vi "MoveBy485.vi"() -> ()   [LabVIEW 2018]
uses:
  <vilib>/robotics/Steering/Create Steering Frame/NI_Robotics_Create Steering Frame.xnode
  <vilib>/robotics/Utilities/Visualization/Steering Visualization/Steering Picture/Draw Steering Frame Options.ctl
  <vilib>/robotics/Steering/Mecanum Steering Frame/NI_Robotics_Mecanum Steering Frame.lvclass
  <vilib>/robotics/Steering/Class Type Definitions/Mecanum Steering Frame.ctl
  XInput9_1_0.dll
  <vilib>/Utility/miscctls.llb/LVPointTypeDef.ctl
  <vilib>/robotics/Steering/Mecanum Steering Frame/Create Mecanum Steering Frame.vi
  <vilib>/robotics/Steering/Mecanum Wheel/Create Mecanum Wheel.vi
  <vilib>/robotics/Steering/Mecanum Wheel/Roller Orientation.ctl
  <vilib>/robotics/Steering/Wheel/Rotation Direction.ctl
  <vilib>/robotics/Steering/Wheel/Wheel Parameters.ctl
  <vilib>/Instr/_visa.llb/VISA Configure Serial Port (Instr).vi
  <vilib>/robotics/Steering/Steering Frame/Apply Steering Frame Velocity to Motors.vi
panel:
  in  "탭 컨트롤":enum32{"Simple", "Setting", "RecipeLab"}(tab)
  out "좌우 속도(m/s)":dbl
  out "회전 속도(rad/s)":dbl
  out "전후 속도(m/s)":dbl
  out "RPM":dbl[](array[numeric])=[0.0, -0.0, 0.0, -0.0]
  in  "Front":bool
  in  "Rear":bool
  in  "Left":bool
  in  "Right":bool
  in  "L Turn":bool
  in  "R Turn":bool
  out "Status":bool
  in  "모터 정지":bool
  out "Motion(Main)":picture caption="Motion"
  in  "최대 전후 속도(m/s)":dbl(slide)=0.1 scale=0.05..0.3
  in  "설정 저장":bool
  in  "최대 좌우 속도(m/s)":dbl(slide)=0.1 scale=0.05..0.3
  in  "최대 회전 속도(rad/s)":dbl(slide)=0.1 scale=0.05..0.3
  in  "RecipeLab 탭 컨트롤":T1(tab)
  in  "Status 유효시간(s)":dbl=0.1
  in  "정지신호 대기시간 (ms)":u32=3000
  out "출력속도(rpm)(recipelab)":dbl[](array[numeric])=[0.0, -0.0, 0.0, -0.0]
  in  "속도제한(rpm)":dbl=2000.0 format="%#_17g"
  in  "속도배율(rpm)":dbl=1.0
  in  "정지":bool
  in  "휠역전":bool[](array[boolean])=[FALSE, FALSE, FALSE, FALSE]
  in  "ID":u8[](array[numeric])=[11, 12, 13, 14]
  in  "Ratio":dbl=50.0 format="%#_13g"
  out "수신 timestamp":timestamp format="%<%H:%M:%S%3u>T"
  out "수신데이터":u8[](array[numeric])
  out "송신데이터":u8[][](array[numeric])
  out "Serial Bytes":u32
  out "송신 timestamp":timestamp=timestamp(3699356400 s since 1904-01-01) format="%<%H:%M:%S%3u>T"
  in  "VISA Write":bool=TRUE
  in  "VISA":refnum<visa-resource-name>="COM7"
  out "송신주기(ms)":u32(graph)=41
  out "수신주기(ms)":u32(graph)
  in  "Angular Velocity (rad/s)":dbl(slide) min=-0.5 max=0.5 step=0.01 scale=-0.1..0.1
  in  "Lateral Velocity (m/s)":dbl(slide) min=-0.5 max=0.5 step=0.01 scale=-0.1..0.1
  in  "Forward Velocity (m/s)":dbl(slide) min=-0.5 max=0.5 step=0.01 scale=-0.1..0.1
  out "Motion(Control)":picture caption="Motion"
  out "출력속도(rpm)(Control)":dbl[](array[numeric])=[0.0, -0.0, 0.0, -0.0]
  out "Buttons":T2
  out "XInput Return":u32
  out "pState":T3
  out "X(Joy)":dbl
  out "Y(Joy)":dbl
  out "Z(Joy)":dbl
  in  "조이스틱 사용":bool
  out "조이스틱 연결됨?":bool
  in  "속도배율(Joy)":dbl=0.05 format="%#_13g"
  out "Motion(Joy)":picture caption="Motion"
  out "출력속도(rpm)(Joystick)":dbl[](array[numeric])=[0.0, -0.0, 0.0, -0.0]
  in  "VISA(str)":string="COM7"
  in  "저장라벨명":string[](array[string])=["저장라벨명", "저장라벨명(str)", "정지신호 대기시간 (ms)", "속도제한(rpm)", "속도배율(rpm)", "휠역전", "VISA Write", "속도배율(Joy)", "ID", "Status 유효시간(s)", "최대 전후 속도(m/s)", "최대 좌우 속도(m/s)", "최대 회전 속도(rad/s)", "Ratio"]
  in  "저장라벨명(str)":string[](array[string])=["VISA(str)"]
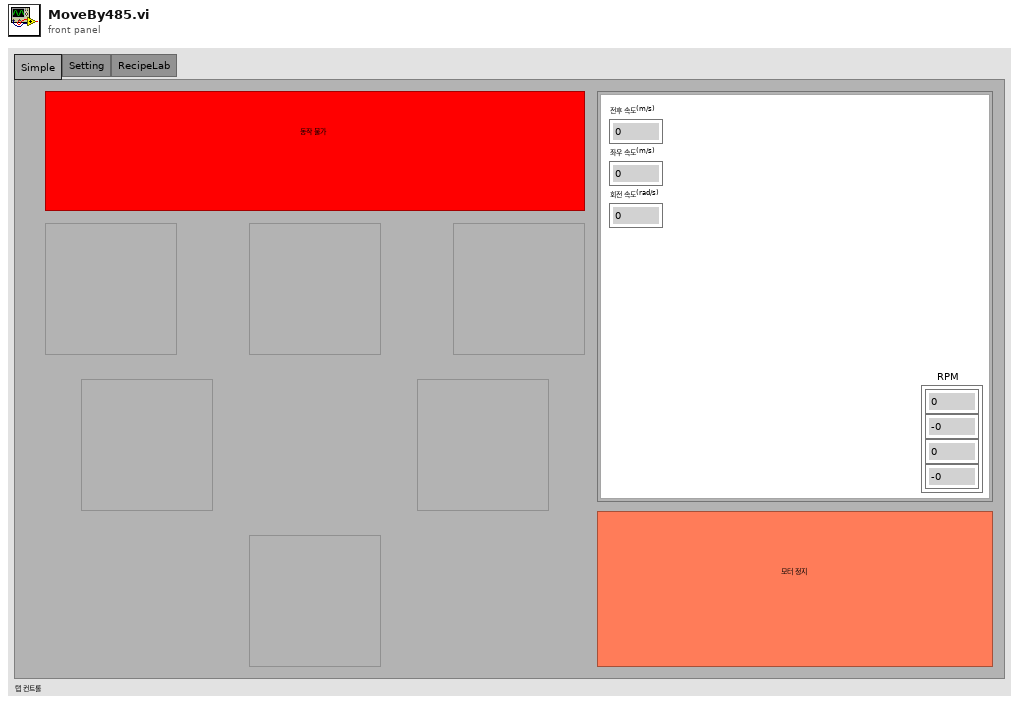
[diagram p1: front panel]
types:
  T1 = enum32{"RecipeLab", "Serial", "Control", "Joystick", "Setting"}
  T2 = cluster{"Dpad Up":bool, "Dpad Down":bool, "Dpad Left":bool, "Dpad Right":bool, "Menu":bool, "View":bool, "L Stick":bool, "R Stick":bool, "L Bumper":bool, "R Bumper":bool, "UNKNOWN":bool, "UNKNOWN":bool, "A":bool, "B":bool, "X":bool, "Y":bool}
  T3 = cluster{"Packet Number":u32, "Gamepad":cluster{"Buttons":u16, "Left Trigger":u8, "Right Trigger":u8, "Thumb LX":i16, "Thumb LY":i16, "Thumb RX":i16, "Thumb RY":i16}}
  T4 = enum32{"invalid app kind", "Development System", "Run Time System", "Student Edition", "Embedded LabVIEW", "Evaluation", "Custom"}
  T5 = typedef "LVPointTypeDef.ctl" = cluster{"Horizontal":i16, "Vertical":i16}
  T6 = cluster{"Boolean array[0]":bool, "Boolean array[1]":bool, "Boolean array[2]":bool, "Boolean array[3]":bool, "Boolean array[4]":bool, "Boolean array[5]":bool, "Boolean array[6]":bool, "Boolean array[7]":bool, "Boolean array[8]":bool, "Boolean array[9]":bool, "Boolean array[10]":bool, "Boolean array[11]":bool, "Boolean array[12]":bool, "Boolean array[13]":bool, "Boolean array[14]":bool, "Boolean array[15]":bool}
  T7 = typedef "NI_Robotics_Steering Picture.lvlib/Draw Steering Frame Options.ctl" = cluster{"draw wheel states?":bool, "highlight wheel index":i32, "pixels per unit":dbl, "draw forward velocity?":bool, "velocity scale":dbl}
  T8 = typedef "LVBoundsTypeDef.ctl" = cluster{"Width":u32, "Height":u32}
  T9 = typedef "NI_Robotics_Steering Class Types.lvlib/Mecanum Steering Frame.ctl" = refnum<class "NI_Robotics_Mecanum Steering Frame.lvclass">
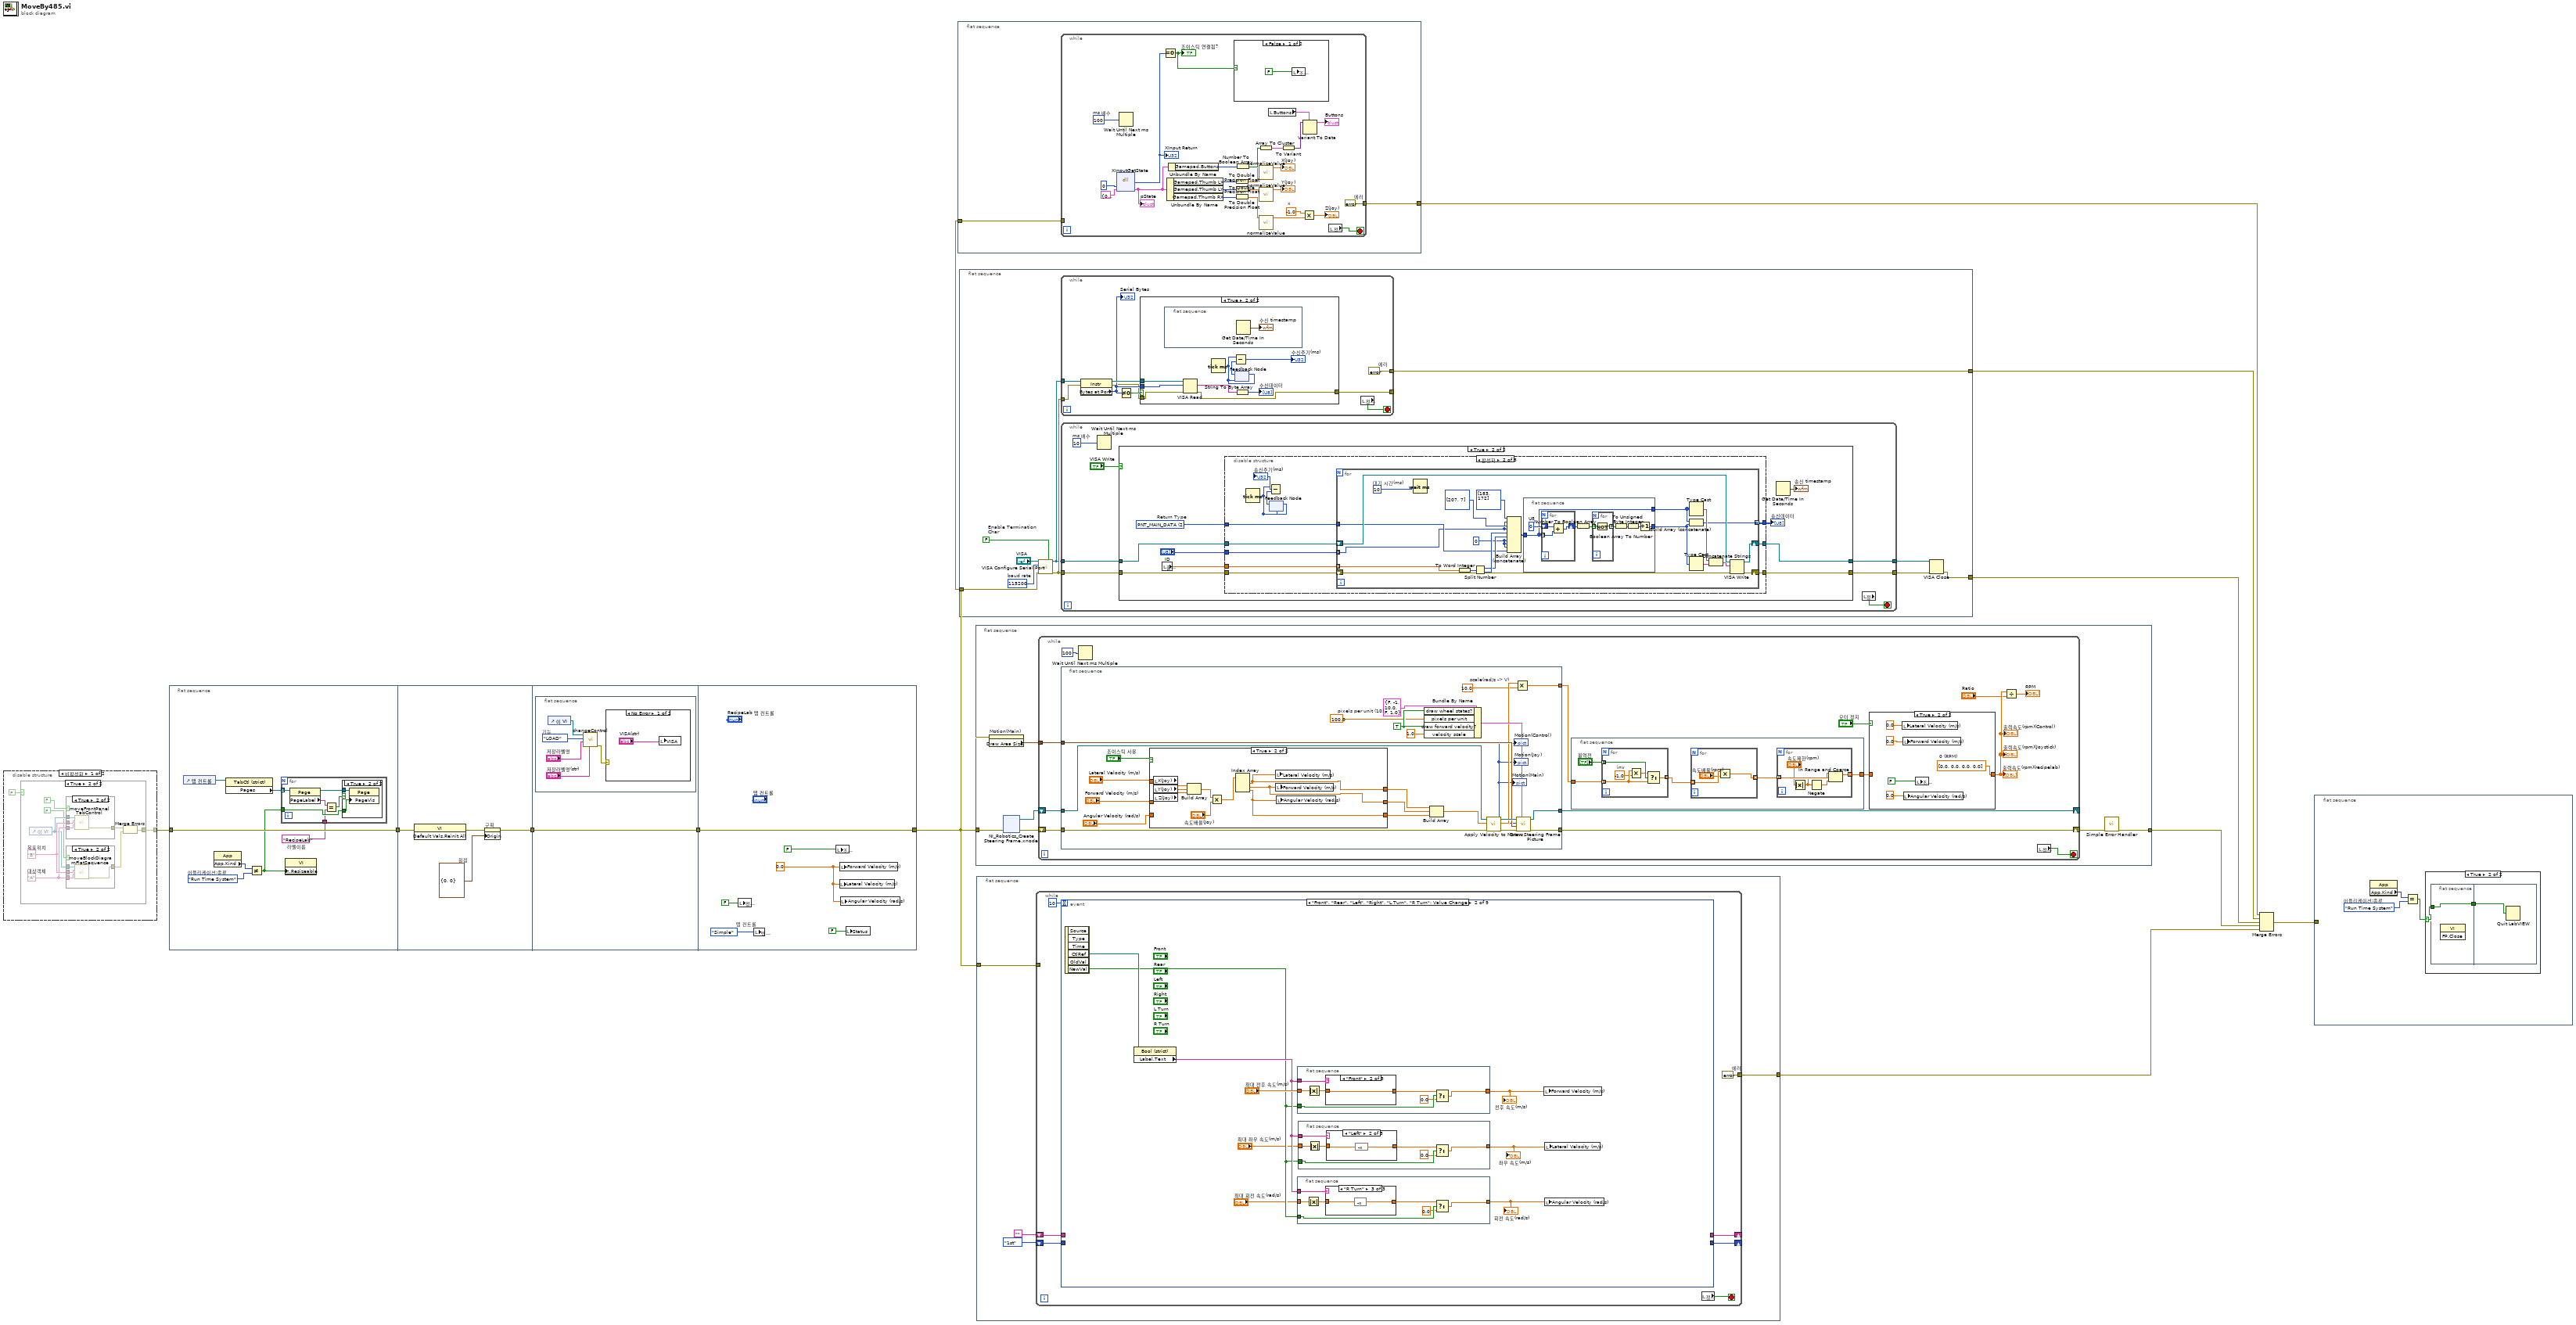
[diagram p0: block diagram]
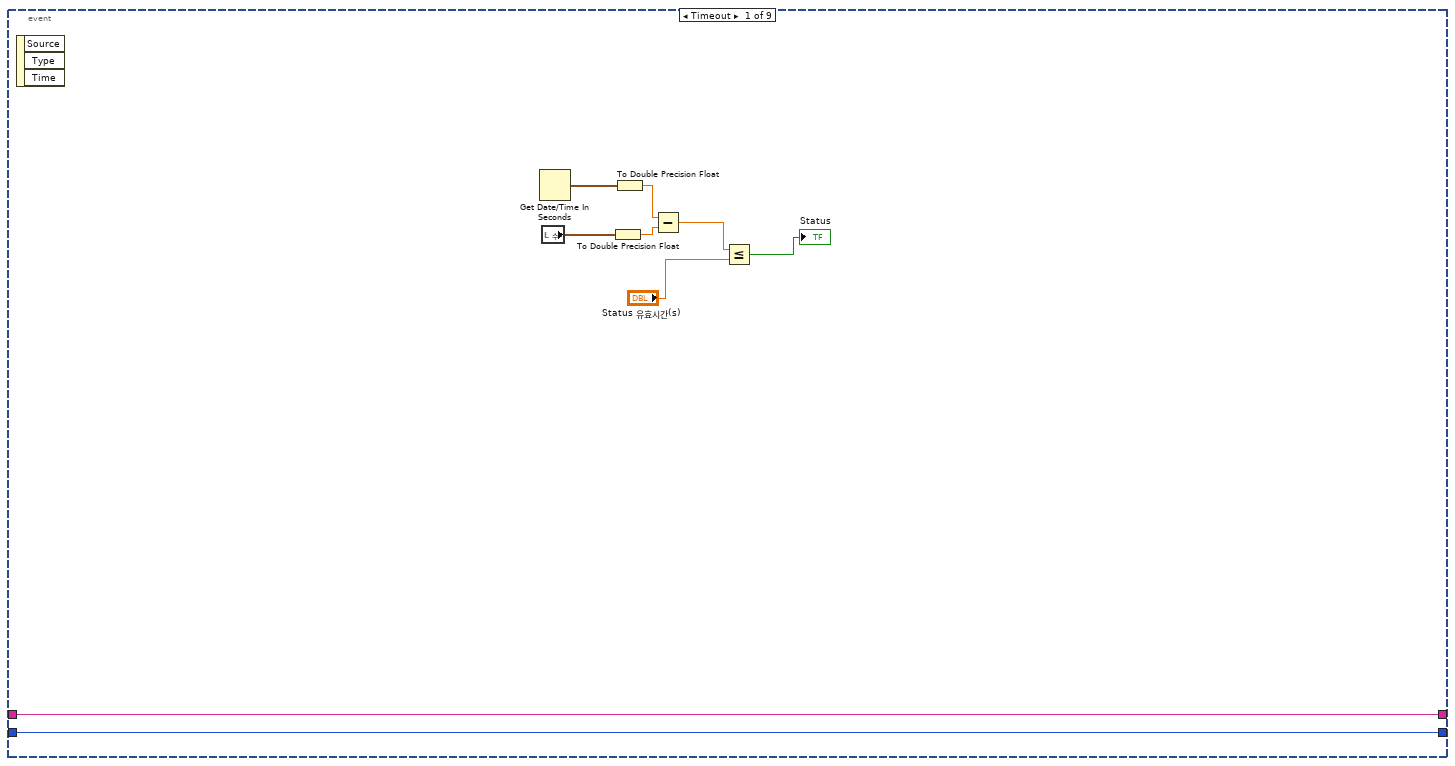
[diagram p2: hidden frame]
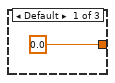
[diagram p3: hidden frame]
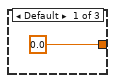
[diagram p5: hidden frame]
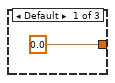
[diagram p7: hidden frame]
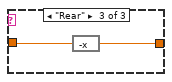
[diagram p8: hidden frame]
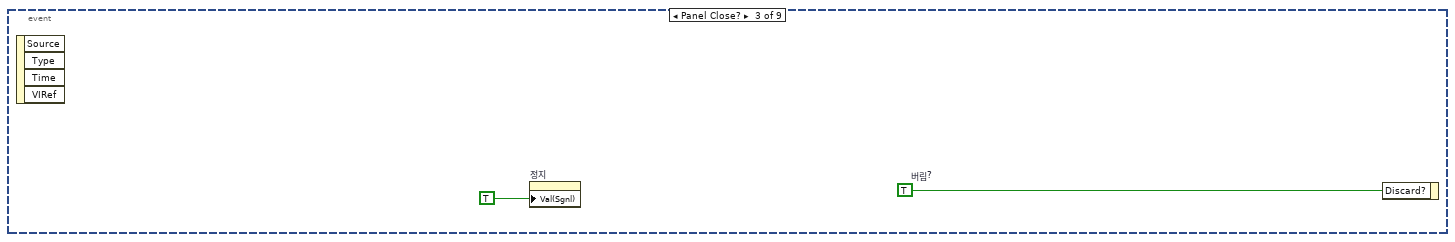
[diagram p9: hidden frame]
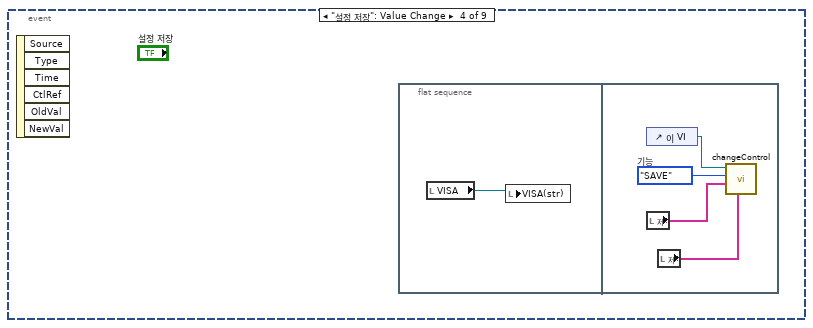
[diagram p10: hidden frame]
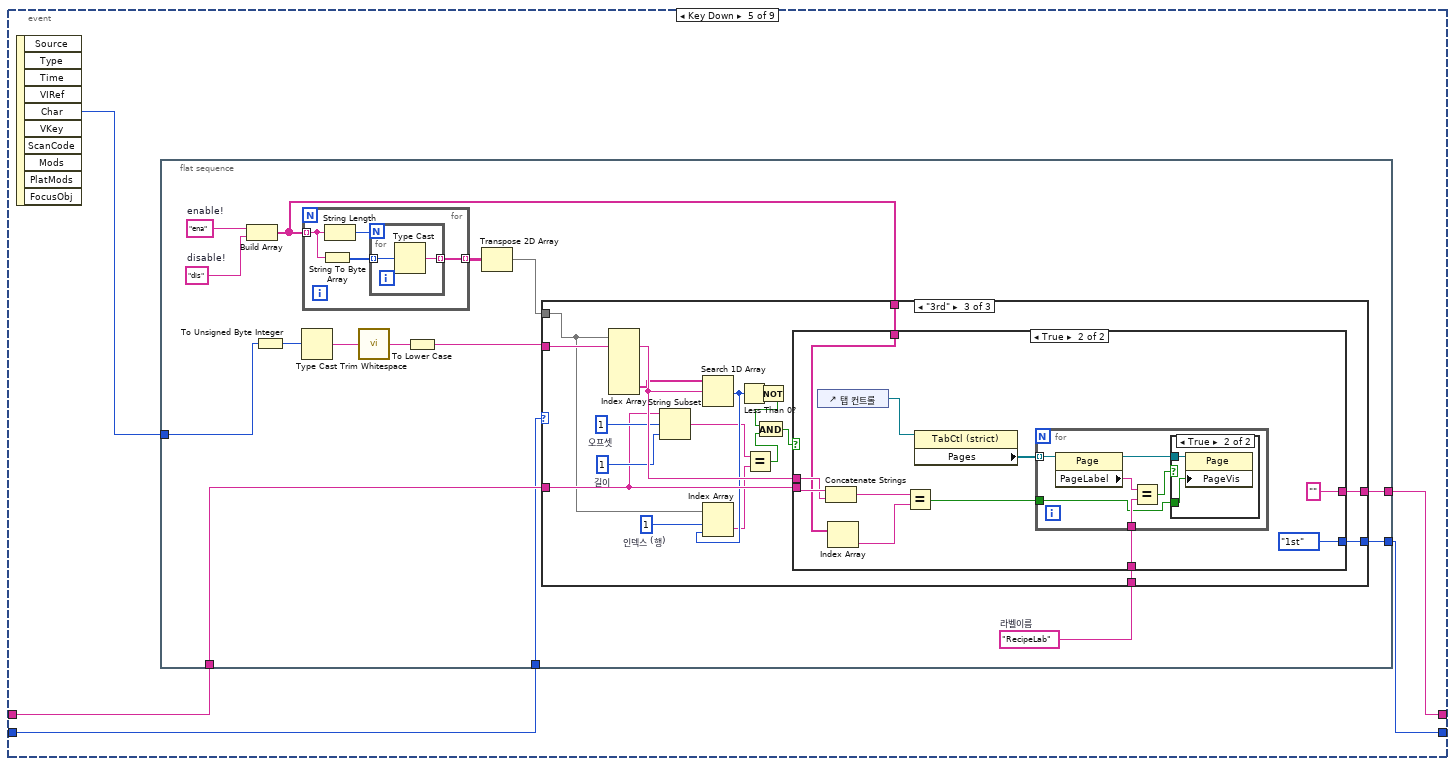
[diagram p11: hidden frame]
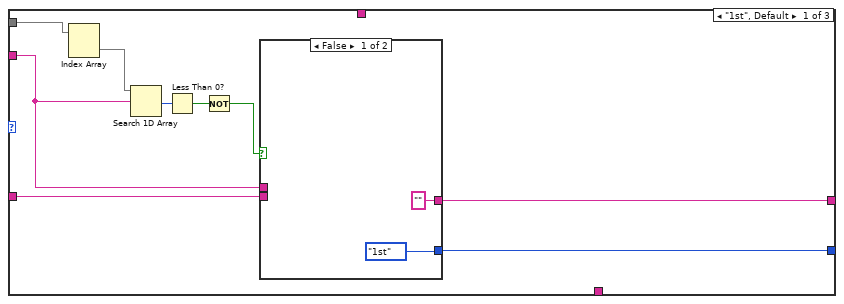
[diagram p12: hidden frame]
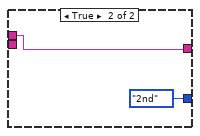
[diagram p13: hidden frame]
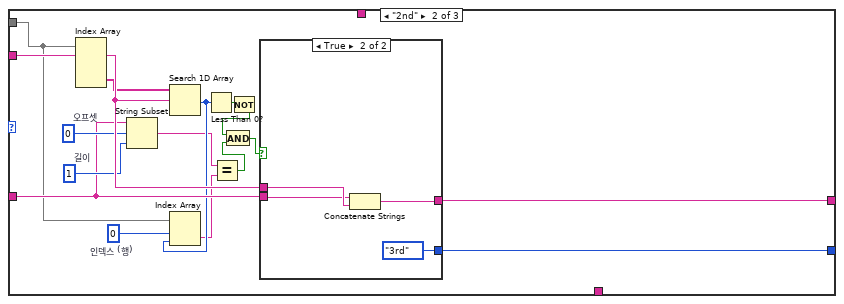
[diagram p14: hidden frame]
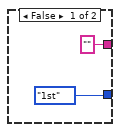
[diagram p15: hidden frame]
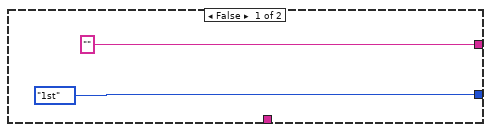
[diagram p16: hidden frame]
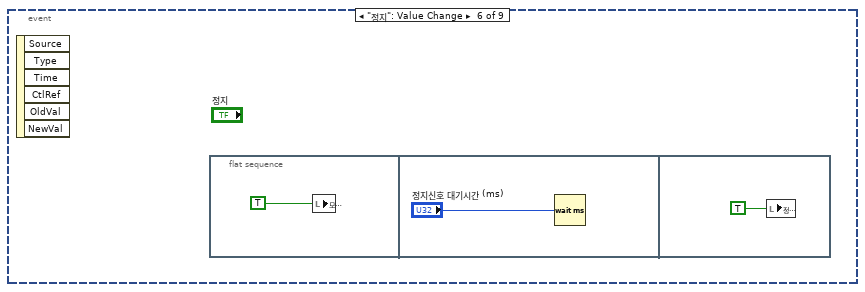
[diagram p18: hidden frame]
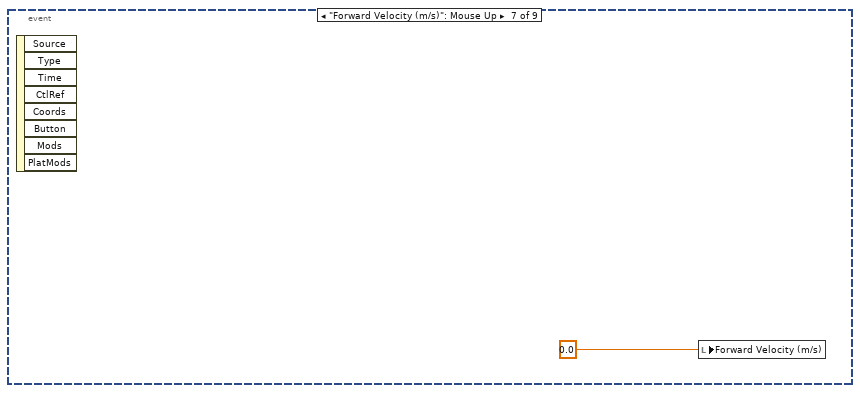
[diagram p19: hidden frame]
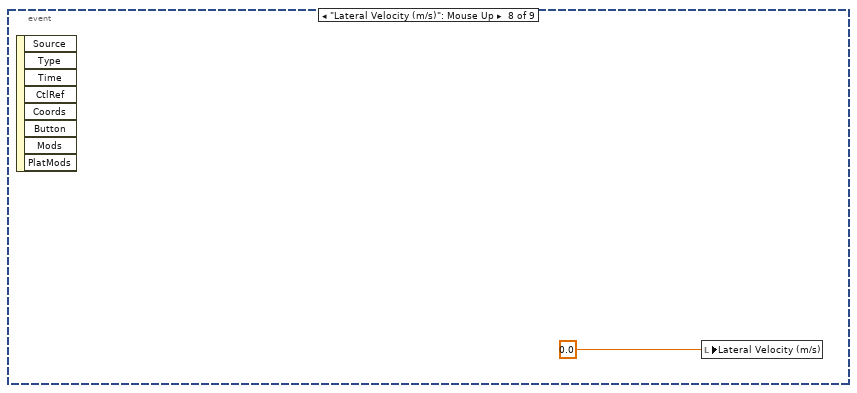
[diagram p20: hidden frame]
diagram:
  n1 = disable-structure shown="비활성화" {
    disable-tunnel: [w12 _] -> w11
    frame Disabled {
      n2 = case shown="True" FALSE {
        tunnel: [_ w14] -> w12
        frame False {
        }
        frame True {
          w20 = "A"  # 대상객체
          w21 = "B"  # 목표위치
          n3 = control-ref of="이 VI"() -> (w19:refnum<vi>)
          n4 = case shown="True" FALSE {
            tunnel: w19 -> [_ w31]
            tunnel: w21 -> [_ w30]
            tunnel: w20 -> [_ w29]
            tunnel: [w27 w28] -> w18
            frame False {
              w27 = errorcluster {"status"=FALSE, "code"=0, "source"=""}  # 에러
            }
            frame True {
              n5 = call "moveFrontPanelTabControl.vi"("대상객체"=w29, "목표위치"=w30, "VI 참조"=w31) -> ("error out"=w28:errorcluster)  [unwired: 7 in, 1 out]
            }
          }
          n6 = case shown="True" FALSE {
            tunnel: w21 -> [_ w26]
            tunnel: w20 -> [_ w25]
            tunnel: w19 -> [_ w24]
            tunnel: [w22 w23] -> w17
            frame False {
              w22 = errorcluster {"status"=FALSE, "code"=0, "source"=""}  # 에러
            }
            frame True {
              n7 = call "moveBlockDiagramFlatSequence.vi"("대상객체"=w25, "목표위치"=w26, "VI 참조"=w24) -> ("error out"=w23:errorcluster)  [unwired: 7 in, 1 out]
            }
          }
          n8 = Merge Errors(w18, w17) -> (w14:errorcluster)
        }
      }
    }
    frame Enabled {
    }
  }
  n9 = flat-sequence {
    tunnel: w11 -> [w38]
    tunnel: [w38] -> w10
    tunnel: [w49] -> w9
    tunnel: w10 -> [w50]
    tunnel: w9 -> [w51]
    tunnel: [w51] -> w8
    tunnel: [w63] -> w3
    tunnel: w8 -> [w63]
    frame #0 {
      w34 = "RecipeLab"  # 라벨이름
      w33 = T4."Run Time System"  # 어플리케이션:종류
      n10 = control-ref of="탭 컨트롤"() -> (w32:refnum<vi>)
      n11 = property class="App"() -> ("App.Kind"=w35:T4)  [unwired: 2 in, 2 out]
      n12 = property class="TabCtl (strict)"(reference=w32) -> ("Pages"=w36:refnum<vi>[])  [unwired: 1 in, 2 out]
      n13 = Not Equal?(x=w35, y=w33) -> (x != y?=w37:bool)
      n14 = for {
        tunnel: w36 -> [w44] mode=indexing
        tunnel: w37 -> [w40]
        tunnel: w34 -> [w39]
        n15 = property class="Page"(reference=w44) -> (reference out=w41:refnum<vi>, "PageLabel"=w43:string)  [unwired: 1 in, 1 out]
        n16 = Equal?(x=w43, y=w39) -> (x = y?=w42:bool)
        n17 = case shown="True" w42 {
          tunnel: w41 -> [_ w46]
          tunnel: w40 -> [_ w45]
          frame False {
          }
          frame True {
            n18 = property class="Page"(reference=w46, "PageVis"=w45) -> ()  [unwired: 1 in, 2 out]
          }
        }
      }
      n19 = property on="프로퍼티 노드" class="VI"("Front Panel.Resizeable"=w37) -> ()  [unwired: 2 in, 2 out]
    }
    frame #1 {
      w48 = T5 {"Horizontal"=0, "Vertical"=0}  # 원점
      n20 = invoke class="VI" method="Default Vals.Reinit All"(error in=w50) -> (error out=w47:errorcluster)  [unwired: 2 in, 2 out]
      n21 = property on="구획" class="Pane"(error in=w47, "Origin"=w48) -> (error out=w49:errorcluster)  [unwired: 1 in, 1 out]
    }
    frame #2 {
      n22 = flat-sequence {
        frame #0 {
          w53 = enum16{"LOAD", "SAVE"}."LOAD"  # 기능
          n23 = control-ref of="이 VI"() -> (w54:refnum<vi>)
          n24 = call "changeControl.vi"("라벨명(str)"="저장라벨명(str)", "라벨명"="저장라벨명", "기능"=w53, "VI 참조"=w54) -> ("error out"=w52:errorcluster)  [unwired: 7 in]
          n25 = case shown="No Error" w52 {
            frame No Error {
              n26 = local write "VISA"("VISA(str)") -> ()
            }
            frame Error {
            }
          }
        }
      }
    }
    frame #3 {
      w59 = 0.0
      w60 = enum32{"Simple", "Setting", "RecipeLab"}."Simple"  # 탭 컨트롤
      n27 = local write "정지"(FALSE) -> ()
      n28 = local write "탭 컨트롤"(w60) -> ()
      n29 = local write "조이스틱 사용"(FALSE) -> ()
      n30 = local write "Lateral Velocity (m/s)"(w59) -> ()
      n31 = local write "Forward Velocity (m/s)"(w59) -> ()
      n32 = local write "Angular Velocity (rad/s)"(w59) -> ()
      n33 = local write "Status"(FALSE) -> ()
    }
  }
  n34 = flat-sequence {
    tunnel: w3 -> [w65]
    tunnel: [w64] -> w7
    frame #0 {
      n35 = while {
        tunnel: w65 -> [_]
        tunnel: [w67] -> w64
        stop <- w73 stop-if-true
        w67 = errorcluster {"status"=FALSE, "code"=0, "source"=""}  # 에러
        w68 = -1.0  # x
        w90 = u32 100  # ms 배수
        n36 = dll-call lib="XInput9_1_0.dll" fn="XInputGetState"("dwUserIndex"=u32 0, "pState"=T3 {"Packet Number"=0, "Gamepad"={"Buttons"=0, "Left Trigger"=0, "Right Trigger"=0, "Thumb LX"=0, "Thumb LY"=0, "Thumb RX"=0, "Thumb RY"=0}} ("XInput State")) -> ("return type"=w82:u32, "pState"=w80:T3)  [unwired: 4 in, 2 out]
        "XInput Return" <- w82
        "pState" <- w80
        n37 = Wait Until Next ms Multiple(millisecond multiple=w90) -> ()  [unwired: 1 out]
        n38 = Equal To 0?(x=w82) -> (x = 0?=w66:bool)
        "조이스틱 연결됨?" <- w66
        n39 = Unbundle By Name(w80) -> ("Gamepad.Thumb LX"=w79:i16, "Gamepad.Thumb LY"=w76:i16, "Gamepad.Thumb RX"=w70:i16)
        n40 = Unbundle By Name(w80) -> ("Gamepad.Buttons"=w85:u16)
        n41 = case shown="False" w66 {
          frame False {
            n42 = local write "조이스틱 사용"(FALSE) -> ()
          }
          frame True {
          }
        }
        n43 = To Double Precision Float(number=w79) -> (double precision float=w78:dbl)
        n44 = To Double Precision Float(number=w76) -> (double precision float=w75:dbl)
        n45 = To Double Precision Float(number=w70) -> (double precision float=w71:dbl)
        n46 = Number To Boolean Array(number=w85) -> (Boolean array=w83:bool[])
        n47 = Array To Cluster(array=w83) -> (cluster=w89:T6)
        n48 = call "normalizeValue.vi"("입력"=w78) -> ("출력"=→"X(Joy)":dbl)  [unwired: 9 in, 1 out]
        n49 = call "normalizeValue.vi"("입력"=w75) -> ("출력"=→"Y(Joy)":dbl)  [unwired: 9 in, 1 out]
        n50 = call "normalizeValue.vi"("입력"=w71) -> ("출력"=w72:dbl)  [unwired: 9 in, 1 out]
        n51 = local read "Buttons"() -> (w84:T2)
        n52 = To Variant(anything=w89) -> (Variant=w88:variant)
        n53 = Multiply(x=w68, y=w72) -> (x*y=→"Z(Joy)":dbl)
        n54 = Variant To Data(type=w84, Variant=w88) -> (data=→"Buttons":T2)  [unwired: 1 in, 1 out]
        n55 = local read "정지"() -> (w73:bool)
      }
    }
  }
  n56 = flat-sequence {
    tunnel: w3 -> [w96]
    tunnel: [w95] -> w6
    tunnel: [w92] -> w2
    frame #0 {
      w99 = FALSE  # Enable Termination Char
      w100 = u32 115200  # baud rate
      n57 = call-poly "VISA Configure Serial Port"("VISA resource name"="VISA", "Enable Termination\nChar (T)"=w99, "baud rate (9600)"=w100, "error in (no error)"=w96) -> ("VISA resource name out"=w97:refnum<visa-resource-name>, "error out"=w98:errorcluster)  [unwired: 10 in]
      n58 = while {
        tunnel: w98 -> [w105]
        tunnel: w97 -> [w109]
        tunnel: [w103] -> _
        tunnel: [w102] -> w95
        stop <- w106 stop-if-true
        w102 = errorcluster {"status"=FALSE, "code"=0, "source"=""}  # 에러
        n59 = property class="Instr"(reference=w109, error in=w105) -> (reference out=w110:refnum<visa-resource-name>, error out=w104:errorcluster, "Bytes at Port"=w107:u32)
        "Serial Bytes" <- w107
        n60 = Not Equal To 0?(x=w107) -> (x != 0?=w108:bool)
        n61 = case shown="True" w108 {
          tunnel: w110 -> [_ w120]
          tunnel: w107 -> [_ w119]
          tunnel: w104 -> [w111 w113]
          tunnel: [w111 w112] -> w103
          frame False {
          }
          frame True {
            n62 = flat-sequence {
              frame #0 {
                n63 = Get Date/Time In Seconds() -> (seconds since 1Jan1904=→"수신 timestamp":timestamp)
              }
            }
            n64 = VISA Read(VISA resource name=w120, byte count=w119, error in (no error)=w113) -> (read buffer=w118:string, error out=w112:errorcluster)  [unwired: 2 out]
            n65 = Tick Count (ms)() -> (millisecond timer value=w115:u32)
            n66 = feedback-in #1(w115) -> ()
            n67 = feedback #1(w115) -> (w116:u32)
            n68 = Subtract(x=w115, y=w116) -> (x-y=→"수신주기(ms)":u32)
            n69 = String To Byte Array(string=w118) -> (unsigned byte array=→"수신데이터":u8[])
          }
        }
        n70 = local read "정지"() -> (w106:bool)
      }
      n71 = while {
        tunnel: w97 -> [w128]
        tunnel: [w124] -> w93
        tunnel: [w123] -> w94
        tunnel: w98 -> [w126]
        stop <- w122 stop-if-true
        w125 = u32 10  # ms 배수
        n72 = Wait Until Next ms Multiple(millisecond multiple=w125) -> ()  [unwired: 1 out]
        n73 = case shown="True" "VISA Write" {
          tunnel: w128 -> [w130 w139]
          tunnel: [w130 w138] -> w124
          tunnel: [w129 w137] -> w123
          tunnel: w126 -> [w129 w136]
          frame False {
          }
          frame True {
            w132 = u8 2 items=["No Return", "PNT_MONITOR", "PNT_MAIN_DATA"]  # Return Type
            n74 = local read "출력속도(rpm)(recipelab)"() -> (w133:dbl[])
            n75 = disable-structure shown="활성화" {
              disable-tunnel: w139 -> [w154 w205 w246]
              disable-tunnel: [w153 w204 w245] -> w138
              disable-tunnel: [w152 w203 w244] -> w137
              disable-tunnel: w136 -> [w151 w202 w243]
              disable-tunnel: "ID" -> [w144 w199 w242]
              disable-tunnel: [w150 w201 w241] -> w134
              disable-tunnel: w133 -> [w143 w200 w240]
              disable-tunnel: w132 -> [w140 w198 _]
              frame Disabled {
                w145 = 2 ("인덱스")
                n76 = Split 1D Array(array=w144, index=w145) -> (first subarray=w146:u8[], second subarray=w147:u8[])
                n77 = Split 1D Array(array=w143, index=w145) -> (first subarray=w148:dbl[], second subarray=w149:dbl[])
                n78 = Build Array(w146, w147) -> (w142:u8[][])
                n79 = Build Array(w148, w149) -> (w141:dbl[][])
                n80 = for {
                  shift-right: [w180] -> w153
                  shift-left: w154 -> [w181]
                  shift-right: [w179] -> w152
                  shift-left: w151 -> [w178]
                  tunnel: w141 -> [w156] mode=indexing
                  tunnel: w142 -> [w157] mode=indexing
                  tunnel: [w173] -> w150 mode=indexing
                  tunnel: w140 -> [w155]
                  w174 = u32 10  # 대기 시간(ms)
                  n81 = Wait (ms)(milliseconds to wait=w174) -> ()  [unwired: 1 out]
                  n82 = Index Array(array=w156) -> (element #1=w166:dbl, element #2=w170:dbl)  [unwired: 2 in]
                  n83 = To Word Integer(number=w166) -> (16bit integer=w165:i16)
                  n84 = To Word Integer(number=w170) -> (16bit integer=w169:i16)
                  n85 = Index Array(array=w157) -> (element #1=w167:u8, element #2=w168:u8)  [unwired: 2 in]
                  n86 = Split Number(x=w165) -> (hi(x)=w162:u8, lo(x)=w163:u8)
                  n87 = Split Number(x=w169) -> (hi(x)=w172:u8, lo(x)=w171:u8)
                  n88 = Build Array (concatenate)(u8[] [183, 172, 254] ("velocity command"), u8[] [207, 7] ("velocity command"), w167, w163, w162, w168, w171, w172, w155) -> (w164:u8[])
                  n89 = flat-sequence {
                    tunnel: [w183] -> w158
                    tunnel: w164 -> [w182]
                    tunnel: [w182] -> w159
                    frame #0 {
                      w189 = u8 0  # U8
                      n90 = for {
                        tunnel: w182 -> [w193] mode=indexing
                        shift-right: [w192] -> w188
                        shift-left: w189 -> [w194]
                        n91 = Add(x=w194, y=w193) -> (x+y=w192:u8)
                      }
                      n92 = Number To Boolean Array(number=w188) -> (Boolean array=w187:bool[])
                      n93 = for {
                        tunnel: w187 -> [w191] mode=indexing
                        tunnel: [w190] -> w186 mode=indexing
                        n94 = Not(x=w191) -> (.not. x?=w190:bool)
                      }
                      n95 = Boolean Array To Number(Boolean array=w186) -> (number=w185:u8)
                      n96 = To Unsigned Byte Integer(number=w185) -> (unsigned 8bit integer=w184:u8)
                      n97 = Increment(x=w184) -> (x+1=w183:u8)
                    }
                  }
                  n98 = Type Cast(x=w159) -> (*(type *) &x=w175:string)  [unwired: 1 in]
                  n99 = Build Array (concatenate)(w159, w158) -> (w173:u8[])
                  n100 = Type Cast(x=w158) -> (*(type *) &x=w177:string)  [unwired: 1 in]
                  n101 = Concatenate Strings(w175, w177) -> (w176:string)
                  n102 = VISA Write(VISA resource name=w181, write buffer=w176, error in (no error)=w178) -> (VISA resource name out=w180:refnum<visa-resource-name>, error out=w179:errorcluster)  [unwired: 1 out]
                }
              }
              frame Enabled {
                n103 = Tick Count (ms)() -> (millisecond timer value=w196:u32)
                n104 = feedback #2(w196) -> (w195:u32)
                n105 = Subtract(x=w196, y=w195) -> (x-y=→"송신주기(ms)":u32)
                n106 = feedback-in #2(w196) -> ()
                n107 = for {
                  shift-right: [w225] -> w204
                  shift-left: w205 -> [w226]
                  shift-right: [w224] -> w203
                  shift-left: w202 -> [w223]
                  tunnel: w200 -> [w208] mode=indexing
                  tunnel: w199 -> [w207] mode=indexing
                  tunnel: [w218] -> w201 mode=indexing
                  tunnel: w198 -> [w209]
                  w206 = u8 0
                  w219 = u32 10  # 대기 시간(ms)
                  n108 = Wait (ms)(milliseconds to wait=w219) -> ()  [unwired: 1 out]
                  n109 = To Word Integer(number=w208) -> (16bit integer=w217:i16)
                  n110 = Split Number(x=w217) -> (hi(x)=w214:u8, lo(x)=w215:u8)
                  n111 = Build Array (concatenate)(u8[] [183, 172] ("velocity command"), w207, u8[] [207, 7] ("velocity command"), w207, w215, w214, w206, w206, w206, w209) -> (w216:u8[])
                  n112 = flat-sequence {
                    tunnel: [w228] -> w210
                    tunnel: w216 -> [w227]
                    tunnel: [w227] -> w211
                    frame #0 {
                      w234 = u8 0  # U8
                      n113 = for {
                        tunnel: w227 -> [w238] mode=indexing
                        shift-right: [w237] -> w233
                        shift-left: w234 -> [w239]
                        n114 = Add(x=w239, y=w238) -> (x+y=w237:u8)
                      }
                      n115 = Number To Boolean Array(number=w233) -> (Boolean array=w232:bool[])
                      n116 = for {
                        tunnel: w232 -> [w236] mode=indexing
                        tunnel: [w235] -> w231 mode=indexing
                        n117 = Not(x=w236) -> (.not. x?=w235:bool)
                      }
                      n118 = Boolean Array To Number(Boolean array=w231) -> (number=w230:u8)
                      n119 = To Unsigned Byte Integer(number=w230) -> (unsigned 8bit integer=w229:u8)
                      n120 = Increment(x=w229) -> (x+1=w228:u8)
                    }
                  }
                  n121 = Type Cast(x=w211) -> (*(type *) &x=w220:string)  [unwired: 1 in]
                  n122 = Build Array (concatenate)(w211, w210) -> (w218:u8[])
                  n123 = Type Cast(x=w210) -> (*(type *) &x=w222:string)  [unwired: 1 in]
                  n124 = Concatenate Strings(w220, w222) -> (w221:string)
                  n125 = VISA Write(VISA resource name=w226, write buffer=w221, error in (no error)=w223) -> (VISA resource name out=w225:refnum<visa-resource-name>, error out=w224:errorcluster)  [unwired: 1 out]
                }
              }
              frame Disabled {
                n126 = for {
                  shift-right: [w264] -> w245
                  shift-left: w246 -> [w265]
                  shift-right: [w263] -> w244
                  shift-left: w243 -> [w262]
                  tunnel: w240 -> [w255] mode=indexing
                  tunnel: w242 -> [w251] mode=indexing
                  tunnel: [w247] -> w241 mode=indexing
                  w250 = u32 10  # 대기 시간(ms)
                  w252 = u8[] [130, 2]  # velocity command
                  w253 = u8[] [183, 172]  # velocity command
                  n127 = To Word Integer(number=w255) -> (16bit integer=w254:i16)
                  n128 = Wait (ms)(milliseconds to wait=w250) -> ()  [unwired: 1 out]
                  n129 = Split Number(x=w254) -> (hi(x)=w259:u8, lo(x)=w258:u8)
                  n130 = Build Array (concatenate)(w253, w251, w252, w258, w259) -> (w257:u8[])
                  n131 = flat-sequence {
                    tunnel: [w267] -> w248
                    tunnel: w257 -> [w266]
                    tunnel: [w266] -> w249
                    frame #0 {
                      w273 = u8 0  # U8
                      n132 = for {
                        tunnel: w266 -> [w277] mode=indexing
                        shift-right: [w276] -> w272
                        shift-left: w273 -> [w278]
                        n133 = Add(x=w278, y=w277) -> (x+y=w276:u8)
                      }
                      n134 = Number To Boolean Array(number=w272) -> (Boolean array=w271:bool[])
                      n135 = for {
                        tunnel: w271 -> [w275] mode=indexing
                        tunnel: [w274] -> w270 mode=indexing
                        n136 = Not(x=w275) -> (.not. x?=w274:bool)
                      }
                      n137 = Boolean Array To Number(Boolean array=w270) -> (number=w269:u8)
                      n138 = To Unsigned Byte Integer(number=w269) -> (unsigned 8bit integer=w268:u8)
                      n139 = Increment(x=w268) -> (x+1=w267:u8)
                    }
                  }
                  n140 = Type Cast(x=w249) -> (*(type *) &x=w256:string)  [unwired: 1 in]
                  n141 = Build Array (concatenate)(w249, w248) -> (w247:u8[])
                  n142 = Type Cast(x=w248) -> (*(type *) &x=w261:string)  [unwired: 1 in]
                  n143 = Concatenate Strings(w256, w261) -> (w260:string)
                  n144 = VISA Write(VISA resource name=w265, write buffer=w260, error in (no error)=w262) -> (VISA resource name out=w264:refnum<visa-resource-name>, error out=w263:errorcluster)  [unwired: 1 out]
                }
              }
            }
            "송신데이터" <- w134
            n145 = Get Date/Time In Seconds() -> (seconds since 1Jan1904=→"송신 timestamp":timestamp)
          }
        }
        n146 = local read "정지"() -> (w122:bool)
      }
      n147 = VISA Close(VISA resource name=w93, error in (no error)=w94) -> (error out=w92:errorcluster)
    }
  }
  n148 = flat-sequence {
    tunnel: w3 -> [w281]
    tunnel: [w279] -> w1
    frame #0 {
      n149 = property on="Motion(Main)" class="Pict"(error in=w281) -> ("Draw Area Size"=w284:T8)  [unwired: 1 in, 2 out]
      n150 = xnode ("NI_Robotics_Create Steering Frame.xnode")("error in (no error)"=w281) -> ("mecanum steering frame out"=w283:T9, "error out"=w282:errorcluster)
      n151 = while {
        shift-right: [w320] -> _
        shift-left: w283 -> [w322]
        shift-right: [w318] -> w280
        shift-left: w282 -> [w321]
        tunnel: w284 -> [w319]
        stop <- w314 stop-if-true
        n152 = flat-sequence {
          tunnel: w322 -> [w352]
          tunnel: w321 -> [w351]
          tunnel: [w350] -> w320
          tunnel: w319 -> [w347]
          tunnel: [w341] -> w318
          tunnel: [w338] -> w317
          frame #0 {
            w343 = 100.0  # pixels per unit (10)
            w339 = 10.0  # scale(rad/s -> V)
            w344 = TRUE ("draw wheel states")
            n153 = case shown="True" "조이스틱 사용" {
              tunnel: [w356 w360] -> w335
              tunnel: "Lateral Velocity (m/s)" -> [w356 _]
              tunnel: [w355 w359] -> w333
              tunnel: "Forward Velocity (m/s)" -> [w355 _]
              tunnel: [w354 w357] -> w331
              tunnel: "Angular Velocity (rad/s)" -> [w354 _]
              frame False {
              }
              frame True {
                n154 = local read "X(Joy)"() -> (w364:dbl)
                n155 = local read "Y(Joy)"() -> (w365:dbl)
                n156 = local read "Z(Joy)"() -> (w358:dbl)
                n157 = Build Array(w364, w365, w358) -> (w363:dbl[])
                n158 = Multiply(x=w363, y="속도배율(Joy)") -> (x*y=w361:dbl[])
                n159 = Index Array(array=w361) -> (element #1=w360:dbl, element #2=w359:dbl, element #3=w357:dbl)  [unwired: 3 in]
                n160 = local write "Lateral Velocity (m/s)"(w360) -> ()
                n161 = local write "Forward Velocity (m/s)"(w359) -> ()
                n162 = local write "Angular Velocity (rad/s)"(w357) -> ()
              }
            }
            n163 = Bundle By Name(cluster=T7 {"draw wheel states?"=FALSE, "highlight wheel index"=-1, "pixels per unit"=10.0, "draw forward velocity?"=FALSE, "velocity scale"=1.0} ("draw options"), "draw wheel states?"=w344, "pixels per unit"=w343, "draw forward velocity?"=w344, "velocity scale"=1.0 ("velocity scale (1)")) -> (w342:T7)
            n164 = Build Array(w335, w333, w331) -> (w353:dbl[])
            n165 = call-poly <vilib>:"Apply Velocity to Motors.vi"("error in (no error)"=w351, "steering frame velocity"=w353, "steering frame in"=w352) -> ("error out"=w348:errorcluster, "ccw motor velocity setpoints"=w340:dbl[], "steering frame out"=w349:T9)  [unwired: 4 in, 2 out]
            n166 = Multiply(x=w340, y=w339) -> (x*y=w338:dbl[])
            n167 = call <vilib>:"Draw Steering Frame Picture.vi"("drawing options"=w342, "error in (no error)"=w348, "picture draw area size (pixels)"=w347, "steering frame in"=w349) -> ("error out"=w341:errorcluster, "picture out"=→"Motion(Main)" →"Motion(Joy)" →"Motion(Control)":picture, "steering frame out"=w350:T9)  [unwired: 5 in]
          }
        }
        n168 = Wait Until Next ms Multiple(millisecond multiple=u32 100) -> ()  [unwired: 1 out]
        n169 = flat-sequence {
          tunnel: w317 -> [w369]
          tunnel: [w368] -> w315
          frame #0 {
            n170 = for {
              tunnel: "휠역전" -> [w378] mode=indexing
              tunnel: w369 -> [w376] mode=indexing
              tunnel: [w375] -> w367 mode=indexing
              w374 = -1.0  # inv
              n171 = Multiply(x=w376, y=w374) -> (x*y=w377:dbl)
              n172 = Select(t=w377, s=w378, f=w376) -> (s? t:f=w375:dbl)
            }
            n173 = for {
              tunnel: w367 -> [w373] mode=indexing
              tunnel: [w372] -> w366 mode=indexing
              n174 = Multiply(x=w373, y="속도배율(rpm)") -> (x*y=w372:dbl)
            }
            n175 = for {
              tunnel: w366 -> [w383] mode=indexing
              tunnel: [w382] -> w368 mode=indexing
              n176 = Absolute Value(x="속도제한(rpm)") -> (abs(x)=w380:dbl)
              n177 = Negate(x=w380) -> (-x=w379:dbl)
              n178 = In Range and Coerce(upper limit=w380, x=w383, lower limit=w379) -> (coerced(x)=w382:dbl)  [unwired: 1 out]
            }
          }
        }
        n179 = case shown="True" "모터 정지" {
          tunnel: [w324 w329] -> w313
          tunnel: w315 -> [w324 _]
          frame False {
          }
          frame True {
            w329 = dbl[] [0.0, 0.0, 0.0, 0.0]  # 0 (RPM)
            n180 = local write "Lateral Velocity (m/s)"(0.0) -> ()
            n181 = local write "Forward Velocity (m/s)"(0.0) -> ()
            n182 = local write "Angular Velocity (rad/s)"(0.0) -> ()
            n183 = local write "조이스틱 사용"(FALSE ("조이스틱 사용")) -> ()
          }
        }
        "출력속도(rpm)(recipelab)" <- w313
        "출력속도(rpm)(Joystick)" <- w313
        "출력속도(rpm)(Control)" <- w313
        n184 = Divide(x=w313, y="Ratio") -> (x/y=→"RPM":dbl[])
        n185 = local read "정지"() -> (w314:bool)
      }
      n186 = call <vilib>:"Simple Error Handler.vi"("error in (no error)"=w280) -> ("error out"=w279:errorcluster)  [unwired: 4 in, 4 out]
    }
  }
  n187 = flat-sequence {
    tunnel: [w387] -> w5
    tunnel: w3 -> [w386]
    frame #0 {
      n188 = while {
        tunnel: w386 -> [_]
        shift-right: [w390] -> _
        shift-left: "" -> [w392]
        shift-right: [w389] -> _
        shift-left: enum16{"1st", "2nd", "3rd"}."1st" -> [w391]
        tunnel: [w388] -> w387
        stop <- w394 stop-if-true
        w388 = errorcluster {"status"=FALSE, "code"=0, "source"=""}  # 에러
        n189 = event shown="[1] \"Front\", \"Rear\", \"Left\", \"Right\", \"L Turn\", \"R Turn\": Value Change" {
          selector: _ -> [_ _ _ _ _ _ _ _ _]
          dyn-events: _ -> [_ _ _ _ _ _ _ _ _]
          timeout: 10 -> [_ _ _ _ _ _ _ _ _]
          tunnel: w392 -> [w403 _ _ _ w456 _ _ _ _]
          tunnel: w391 -> [w402 _ _ _ w455 _ _ _ _]
          tunnel: [w403 _ _ _ w454 _ _ _ _] -> w390
          tunnel: [w402 _ _ _ w453 _ _ _ _] -> w389
          event Timeout {
            n190 = event-data() -> ()  [unwired: 1 in, 3 out]
            n191 = Get Date/Time In Seconds() -> (seconds since 1Jan1904=w401:timestamp)
            n192 = local read "수신 timestamp"() -> (w400:timestamp)
            n193 = To Double Precision Float(number=w400) -> (double precision float=w398:dbl)
            n194 = To Double Precision Float(number=w401) -> (double precision float=w399:dbl)
            n195 = Subtract(x=w399, y=w398) -> (x-y=w397:dbl)
            n196 = Less Or Equal?(x=w397, y="Status 유효시간(s)") -> (x <= y?=→"Status":bool)
          }
          event "Front", "Rear", "Left", "Right", "L Turn", "R Turn": Value Change {
            n197 = event-data() -> ("CtlRef"=w412:refnum<vi>, "NewVal"=w406:bool)  [unwired: 1 in, 4 out]
            n198 = property class="Bool (strict)"(reference=w412) -> ("Label.Text"=w407:string)  [unwired: 1 in, 2 out]
            n199 = flat-sequence {
              tunnel: w407 -> [w419]
              tunnel: "최대 회전 속도(rad/s)" -> [w418]
              tunnel: [w414] -> w408
              tunnel: w406 -> [w416]
              frame #0 {
                n200 = Absolute Value(x=w418) -> (abs(x)=w417:dbl)
                n201 = case shown="\"R Turn\"" w419 {
                  tunnel: w417 -> [_ w421 w423]
                  tunnel: [0.0 w421 w422] -> w415
                  frame Default {
                  }
                  frame "L Turn" {
                  }
                  frame "R Turn" {
                    n202 = expression code="-x"(w423) -> (w422:dbl)
                  }
                }
                n203 = Select(t=w415, s=w416, f=0.0) -> (s? t:f=w414:dbl)
              }
            }
            n204 = flat-sequence {
              tunnel: w407 -> [w441]
              tunnel: "최대 전후 속도(m/s)" -> [w440]
              tunnel: [w436] -> w410
              tunnel: w406 -> [w438]
              frame #0 {
                n205 = Absolute Value(x=w440) -> (abs(x)=w439:dbl)
                n206 = case shown="\"Front\"" w441 {
                  tunnel: w439 -> [_ w443 w445]
                  tunnel: [0.0 w443 w444] -> w437
                  frame Default {
                  }
                  frame "Front" {
                  }
                  frame "Rear" {
                    n207 = expression code="-x"(w445) -> (w444:dbl)
                  }
                }
                n208 = Select(t=w437, s=w438, f=0.0) -> (s? t:f=w436:dbl)
              }
            }
            n209 = flat-sequence {
              tunnel: w407 -> [w430]
              tunnel: "최대 좌우 속도(m/s)" -> [w429]
              tunnel: [w425] -> w409
              tunnel: w406 -> [w427]
              frame #0 {
                n210 = Absolute Value(x=w429) -> (abs(x)=w428:dbl)
                n211 = case shown="\"Left\"" w430 {
                  tunnel: w428 -> [_ w433 w434]
                  tunnel: [0.0 w432 w434] -> w426
                  frame Default {
                  }
                  frame "Left" {
                    n212 = expression code="-x"(w433) -> (w432:dbl)
                  }
                  frame "Right" {
                  }
                }
                n213 = Select(t=w426, s=w427, f=0.0) -> (s? t:f=w425:dbl)
              }
            }
            n214 = local write "Forward Velocity (m/s)"(w410) -> ()
            n215 = local write "Angular Velocity (rad/s)"(w408) -> ()
            n216 = local write "Lateral Velocity (m/s)"(w409) -> ()
            "전후 속도(m/s)" <- w410
            "좌우 속도(m/s)" <- w409
            "회전 속도(rad/s)" <- w408
          }
          event Panel Close? {
            w447 = TRUE  # 버림?
            n217 = event-data() -> ()  [unwired: 1 in, 4 out]
            n218 = property on="정지" class="Bool (strict)"("Val(Sgnl)"=TRUE) -> ()  [unwired: 2 in, 2 out]
            n219 = event-data("Discard?"=w447) -> ()  [unwired: 1 in, 1 out]
          }
          event "설정 저장": Value Change {
            n220 = event-data() -> ()  [unwired: 1 in, 6 out]
            n221 = flat-sequence {
              frame #0 {
                n222 = local read "VISA"() -> (w448:refnum<visa-resource-name>)
                n223 = local write "VISA(str)"(w448) -> ()
              }
              frame #1 {
                w451 = enum16{"LOAD", "SAVE"}."SAVE"  # 기능
                n224 = control-ref of="이 VI"() -> (w452:refnum<vi>)
                n225 = local read "저장라벨명"() -> (w449:string[])
                n226 = local read "저장라벨명(str)"() -> (w450:string[])
                n227 = call "changeControl.vi"("라벨명(str)"=w450, "라벨명"=w449, "기능"=w451, "VI 참조"=w452) -> ()  [unwired: 7 in, 1 out]
              }
            }
          }
          event Key Down {
            n228 = event-data() -> ("Char"=w457:i16)  [unwired: 1 in, 9 out]
            n229 = flat-sequence {
              tunnel: w457 -> [w468]
              tunnel: w456 -> [w467]
              tunnel: w455 -> [w466]
              tunnel: [w465] -> w454
              tunnel: [w458] -> w453
              frame #0 {
                w459 = "RecipeLab"  # 라벨이름
                w463 = "dis"  # disable!
                w464 = "ena"  # enable!
                n230 = Build Array(w464, w463) -> (w460:string[])
                n231 = To Unsigned Byte Integer(number=w468) -> (unsigned 8bit integer=w470:u8)
                n232 = Type Cast(x=w470) -> (*(type *) &x=w469:string)  [unwired: 1 in]
                n233 = for {
                  tunnel: w460 -> [w475] mode=indexing
                  tunnel: [w473] -> w462 mode=indexing
                  n234 = String To Byte Array(string=w475) -> (unsigned byte array=w474:u8[])
                  n235 = String Length(string=w475) -> (length=w476:i32)
                  n236 = for {
                    N: w476 -> [_]
                    tunnel: w474 -> [w478] mode=indexing
                    tunnel: [w477] -> w473 mode=indexing
                    n237 = Type Cast(x=w478) -> (*(type *) &x=w477:string)  [unwired: 1 in]
                  }
                }
                n238 = call <vilib>:"Trim Whitespace.vi"("string"=w469) -> ("trimmed string"=w471:string)  [unwired: 1 in]
                n239 = To Lower Case(string=w471) -> (all lower case string=w472:string)
                n240 = Transpose 2D Array(2D array=w462) -> (transposed array=w461:string[][])
                n241 = case shown="\"3rd\"" w466 {
                  tunnel: w472 -> [w480 w505 w529]
                  tunnel: w467 -> [w484 w501 w526]
                  tunnel: [w487 w507 w531] -> w465
                  tunnel: [w486 w506 w530] -> w458
                  tunnel: w461 -> [w483 w500 w525]
                  tunnel: w460 -> [_ _ w515]
                  tunnel: w459 -> [_ _ w514]
                  frame "1st", Default {
                    n242 = Index Array(array=w483) -> (element=w485:string[])  [unwired: 2 in]
                    n243 = Search 1D Array(1D array=w485, element=w480) -> (index of element=w482:i32)  [unwired: 1 in]
                    n244 = Less Than 0?(x=w482) -> (x < 0?=w481:bool)
                    n245 = Not(x=w481) -> (.not. x?=w479:bool)
                    n246 = case shown="False" w479 {
                      tunnel: w484 -> [_ _]
                      tunnel: ["" w490] -> w487
                      tunnel: [enum16{"1st", "2nd", "3rd"}."1st" enum16{"1st", "2nd", "3rd"}."2nd"] -> w486
                      tunnel: w480 -> [_ w490]
                      frame False {
                      }
                      frame True {
                      }
                    }
                  }
                  frame "2nd" {
                    w499 = 0  # 인덱스 (행)
                    w502 = 0  # 오프셋
                    w503 = 1  # 길이
                    n247 = Index Array(array=w500) -> (element #2=w504:string[])  [unwired: 4 in, 1 out]
                    n248 = String Subset(string=w501, offset (0)=w502, length (rest)=w503) -> (substring=w497:string)
                    n249 = Search 1D Array(1D array=w504, element=w505) -> (index of element=w498:i32)  [unwired: 1 in]
                    n250 = Index Array(array=w500, index (row)=w499, index (col)=w498) -> (element=w496:string)
                    n251 = Less Than 0?(x=w498) -> (x < 0?=w495:bool)
                    n252 = Equal?(x=w497, y=w496) -> (x = y?=w494:bool)
                    n253 = Not(x=w495) -> (.not. x?=w492:bool)
                    n254 = And(x=w492, y=w494) -> (x .and. y?=w493:bool)
                    n255 = case shown="True" w493 {
                      tunnel: w501 -> [_ w511]
                      tunnel: ["" w510] -> w507
                      tunnel: [enum16{"1st", "2nd", "3rd"}."1st" enum16{"1st", "2nd", "3rd"}."3rd"] -> w506
                      tunnel: w505 -> [_ w512]
                      frame False {
                      }
                      frame True {
                        n256 = Concatenate Strings(w511, w512) -> (w510:string)
                      }
                    }
                  }
                  frame "3rd" {
                    w524 = 1  # 인덱스 (행)
                    w527 = 1  # 오프셋
                    w528 = 1  # 길이
                    n257 = Index Array(array=w525) -> (element #3=w516:string[])  [unwired: 6 in, 2 out]
                    n258 = String Subset(string=w526, offset (0)=w527, length (rest)=w528) -> (substring=w522:string)
                    n259 = Search 1D Array(1D array=w516, element=w529) -> (index of element=w523:i32)  [unwired: 1 in]
                    n260 = Index Array(array=w525, index (row)=w524, index (col)=w523) -> (element=w521:string)
                    n261 = Less Than 0?(x=w523) -> (x < 0?=w520:bool)
                    n262 = Equal?(x=w522, y=w521) -> (x = y?=w519:bool)
                    n263 = Not(x=w520) -> (.not. x?=w517:bool)
                    n264 = And(x=w517, y=w519) -> (x .and. y?=w518:bool)
                    n265 = case shown="True" w518 {
                      tunnel: w526 -> [_ w542]
                      tunnel: ["" ""] -> w531
                      tunnel: [enum16{"1st", "2nd", "3rd"}."1st" enum16{"1st", "2nd", "3rd"}."1st"] -> w530
                      tunnel: w529 -> [_ w541]
                      tunnel: w515 -> [_ w539]
                      tunnel: w514 -> [_ w536]
                      frame False {
                      }
                      frame True {
                        n266 = control-ref of="탭 컨트롤"() -> (w534:refnum<vi>)
                        n267 = Concatenate Strings(w542, w541) -> (w540:string)
                        n268 = Index Array(array=w539) -> (element=w538:string)  [unwired: 1 in]
                        n269 = Equal?(x=w540, y=w538) -> (x = y?=w535:bool)
                        n270 = property class="TabCtl (strict)"(reference=w534) -> ("Pages"=w537:refnum<vi>[])  [unwired: 1 in, 2 out]
                        n271 = for {
                          tunnel: w537 -> [w550] mode=indexing
                          tunnel: w536 -> [w548]
                          tunnel: w535 -> [w545]
                          n272 = property class="Page"(reference=w550) -> (reference out=w546:refnum<vi>, "PageLabel"=w549:string)  [unwired: 1 in, 1 out]
                          n273 = Equal?(x=w549, y=w548) -> (x = y?=w547:bool)
                          n274 = case shown="True" w547 {
                            tunnel: w546 -> [_ w552]
                            tunnel: w545 -> [_ w551]
                            frame False {
                            }
                            frame True {
                              n275 = property class="Page"(reference=w552, "PageVis"=w551) -> ()  [unwired: 1 in, 2 out]
                            }
                          }
                        }
                      }
                    }
                  }
                }
              }
            }
          }
          event "정지": Value Change {
            n276 = event-data() -> ()  [unwired: 1 in, 6 out]
            n277 = flat-sequence {
              frame #0 {
                n278 = local write "모터 정지"(TRUE) -> ()
              }
              frame #1 {
                n279 = Wait (ms)(milliseconds to wait="정지신호 대기시간 (ms)") -> ()  [unwired: 1 out]
              }
              frame #2 {
                n280 = local write "정지"(TRUE) -> ()
              }
            }
          }
          event "Forward Velocity (m/s)": Mouse Up {
            n281 = event-data() -> ()  [unwired: 1 in, 8 out]
            n282 = local write "Forward Velocity (m/s)"(0.0) -> ()
          }
          event "Lateral Velocity (m/s)": Mouse Up {
            n283 = event-data() -> ()  [unwired: 1 in, 8 out]
            n284 = local write "Lateral Velocity (m/s)"(0.0) -> ()
          }
          event "Angular Velocity (rad/s)": Mouse Up {
            n285 = event-data() -> ()  [unwired: 1 in, 8 out]
            n286 = local write "Angular Velocity (rad/s)"(0.0) -> ()
          }
        }
        n287 = local read "정지"() -> (w394:bool)
      }
    }
  }
  n288 = Merge Errors(w7, w6, w2, w1, w5) -> (w4:errorcluster)
  n289 = flat-sequence {
    tunnel: w4 -> [_]
    frame #0 {
      w559 = T4."Run Time System"  # 어플리케이션:종류
      n290 = property class="App"() -> ("App.Kind"=w561:T4)  [unwired: 2 in, 2 out]
      n291 = Equal?(x=w561, y=w559) -> (x = y?=w560:bool)
      n292 = case shown="True" w560 {
        selector: w560 -> [_ w562]
        frame False {
        }
        frame True {
          n293 = flat-sequence {
            tunnel: w562 -> [w564]
            tunnel: [w564] -> w563
            tunnel: w563 -> [w565]
            frame #0 {
              n294 = invoke class="VI" method="FP.Close"() -> ()  [unwired: 3 in, 3 out]
            }
            frame #1 {
              n295 = Quit LabVIEW(quit? (T)=w565) -> ()
            }
          }
        }
      }
    }
  }
